vi "status of worker2.vi"() -> ()   [LabVIEW 2020]
panel:
  out "worker2_busy/ready":bool
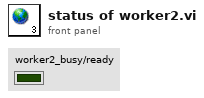
[diagram p1: front panel]
diagram:
